vi "Move Relative Command SubVi.vi"(3 "TargetDisplacement in":dbl[](array[numeric]), 4 "GroupName":string, 5 "error in":errorcluster, 6 "reference in":refnum<k24>) -> (0 "TargetDisplacement out":dbl[](array[numeric]), 1 "error out":errorcluster, 2 "reference out":refnum<k24>)   [LabVIEW 2017]
uses:
  Newport.XPS.CommandInterface
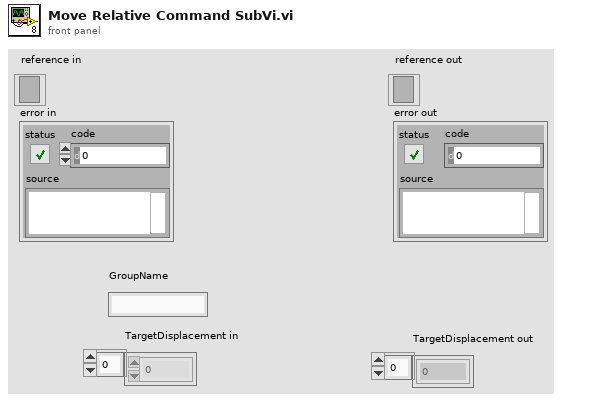
[diagram p1: front panel]
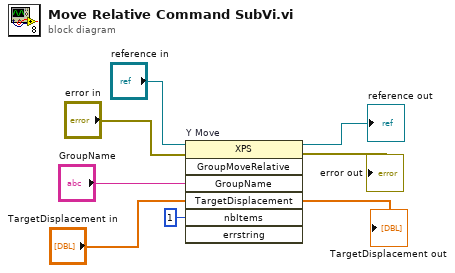
[diagram p0: block diagram]
diagram:
  n1 = invoke on="Y Move" class="XPS" method="GroupMoveRelative"(reference="reference in", error in="error in", "GroupName"="GroupName", "TargetDisplacement"="TargetDisplacement in", "nbItems"=1) -> (reference out=→"reference out":refnum<k24>, error out=→"error out":errorcluster, "TargetDisplacement"=→"TargetDisplacement out":dbl[])  [unwired: 2 in, 4 out]
